vi "generator.vi"() -> ()   [LabVIEW 2018]
panel:
  in  "Uwe":dbl
  in  "czêstotliwoœæ":dbl
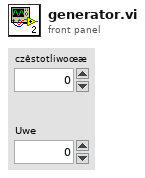
[diagram p1: front panel]
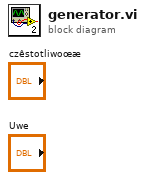
[diagram p0: block diagram]
diagram:
